vi "Switch status IO.vi"(6 "mode":enum16{"READ", "WRITE"}(ring), 8 "error in (no error)":errorcluster, 10 "Channels in":T1=[{"Channel x"="xA1", "Channel y"="yA7"}, {"Channel x"="comD7", "Channel y"="chD7"}, {"Channel x"="comC1", "Channel y"="chC1"}], 11 "Path":path=path "C:/LabView/PPMS basic VIs/Pickering_Switch_Memory.txt") -> (0 "error out":errorcluster, 2 "Channels out":T1, 3 "Path out":path)   [LabVIEW 2016, in "pickering.lvclass"]
uses:
  pickering.lvclass
  Typedefs/Channels-Array.ctl
  Typedefs/Channel-Cluster.ctl
  Typedefs/ChannelX-ComboBox.ctl
  Typedefs/ChannelY-ComboBox.ctl
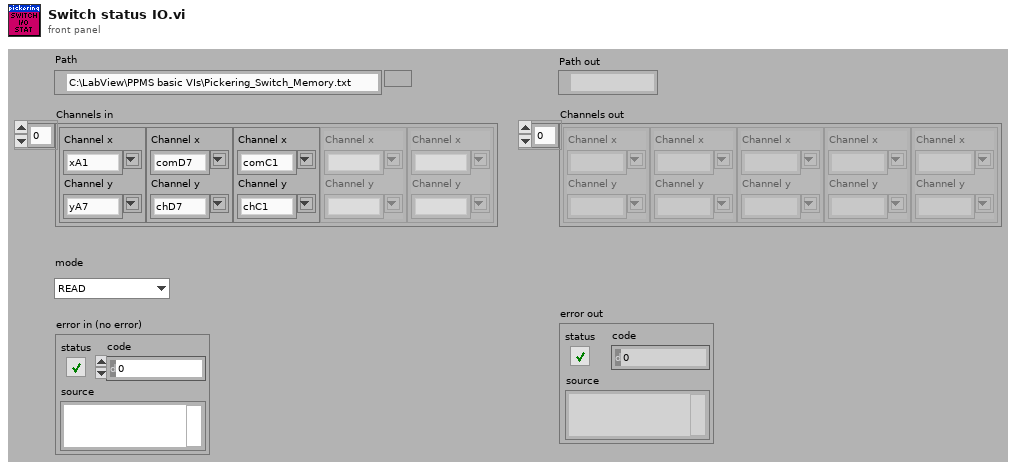
[diagram p1: front panel]
types:
  T1 = typedef "pickering.lvclass/Channels-Array.ctl" = T2[]
  T2 = typedef "pickering.lvclass/Channel-Cluster.ctl" = cluster{"Channel x":T3, "Channel y":T4}
  T3 = typedef "pickering.lvclass/ChannelX-ComboBox.ctl" = string
  T4 = typedef "pickering.lvclass/ChannelY-ComboBox.ctl" = string
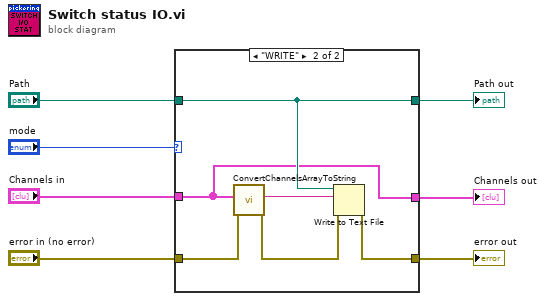
[diagram p0: block diagram]
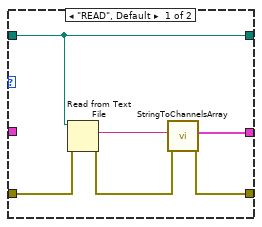
[diagram p2: hidden frame]
diagram:
  n1 = case shown="\"WRITE\"" "mode" {
    tunnel: "Path" -> [w8 w15]
    tunnel: [w8 w15] -> w5
    tunnel: "error in (no error)" -> [w12 w16]
    tunnel: [w9 w18] -> w3
    tunnel: "Channels in" -> [_ w14]
    tunnel: [w11 w14] -> w1
    frame "READ", Default {
      n2 = Read from Text File(file (use dialog)=w8, error in=w12) -> (text=w13:string, error out=w10:errorcluster)  [unwired: 2 in, 2 out]
      n3 = call "StringToChannelsArray.vi"("error in (no error)"=w10, "String"=w13) -> ("error out"=w9:errorcluster, "Array"=w11:T2[])  [unwired: 8 in]
    }
    frame "WRITE" {
      n4 = call "ConvertChannelsArrayToString.vi"("error in (no error)"=w16, "Channels in"=w14) -> ("error out"=w17:errorcluster, "String"=w19:string)  [unwired: 8 in]
      n5 = Write to Text File(file (use dialog)=w15, text=w19, error in=w17) -> (error out=w18:errorcluster)  [unwired: 1 in, 2 out]
    }
  }
  "Path out" <- w5
  "error out" <- w3
  "Channels out" <- w1
